vi "Start.vi"(11 "Custom Device in":refnum<class "NIDMM Engine.lvclass">) -> (0 "error out":errorcluster, 3 "Custom Device out":refnum<class "NIDMM Engine.lvclass">)   [LabVIEW 2026, in "NIDMM Engine.lvlib" / "NIDMM Engine.lvclass"]
uses:
  NIDMM Engine.lvclass
  NIDMM Engine.lvclass/NIDMM Engine.ctl
  <userlib>/NIVS Inline Async API (Express)/_VS Inline Async API (Express)/VS Inline Async API (Express)/VS Inline Async API (Express).lvclass
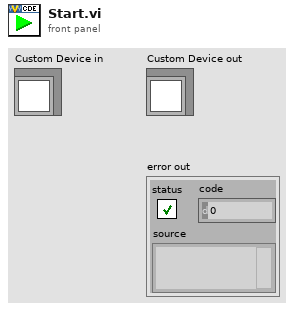
[diagram p1: front panel]
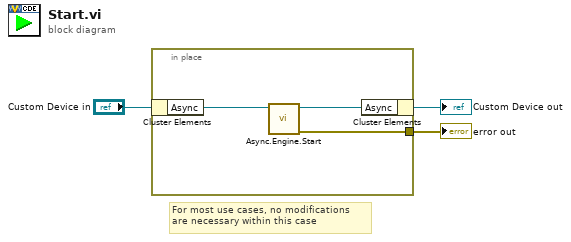
[diagram p0: block diagram]
diagram:
  # "For most use cases, no modifications \nare necessary within this case"
  n1 = in-place {
    in-place-border: [w4] -> w1
    n2 = in-place-cluster #1("Custom Device in") -> ("Async"=w6:refnum<class "VS Inline Async API (Express).lvclass">)
    n3 = call <userlib>:"Async.Engine.Start.vi"("Async in"=w6) -> ("error out"=w4:errorcluster, "Async out"=w5:refnum<class "VS Inline Async API (Express).lvclass">)  [unwired: 9 in]
    n4 = in-place-cluster #1("Async"=w5) -> (→"Custom Device out":refnum<class "NIDMM Engine.lvclass">)
  }
  "error out" <- w1
